vi "Imageprocessing_subVi.vi"(8 "error in (no error)":errorcluster, 10 "Binary Img":T1, 11 "Image In":T1) -> (0 "error out":errorcluster, 3 "Image Dst Out":T1)   [LabVIEW 2020]
doc: "Vi che stima i parametri di calibrazione da un set up specifico (inserire descriz setup!!!).\nCostanti inteerne: Inserire descrizione"
uses:
  <vilib>/vision/Image Controls.llb/IMAQ Image.ctl
  <vilib>/vision/NI_Vision_Development_Module.lvlib
panel:
  in  "stop":bool
  in  "Window Size (32x32)":cluster{"SizeX":i32, "SizeY":i32}={"SizeX"=200, "SizeY"=200}
  in  "Selection Values":T3(array[cluster])=[{"Measurement Parameter"=35, "Range Lower Value"=0.0, "Range Upper Value"=100.0, "Range"=FALSE, "Measurement Type"=FALSE}] {"Measurement Parameter" items=["Center of Mass X", "Center of Mass Y", "First Pixel X", "First Pixel Y", "Bounding Rect Left", "Bounding Rect Top", "Bounding Rect Right", "Bounding Rect Bottom", "Max Feret Diameter Start X", "Max Feret Diameter Start Y", "Max Feret Diameter End X", "Max Feret Diameter End Y", "Max Horiz. Segment Length Left", "Max Horiz. Segment Length Right", "Max Horiz. Segment Length Row", "-", "Bounding Rect Width", "Bounding Rect Height", "Bounding Rect Diagonal", "Perimeter", "Convex Hull Perimeter", "Holes' Perimeter", "Max Feret Diameter", "Equivalent Ellipse Major Axis", "Equivalent Ellipse Minor Axis", "Equivalent Ellipse Minor Axis (Feret)", "Equivalent Rect Long Side", "Equivalent Rect Short Side", "Equivalent Rect Diagonal", "Equivalent Rect Short Side (Feret)", "Average Horiz. Segment Length", "Average Vert. Segment Length", "Hydraulic Radius", "Waddel Disk Diameter", "-", "Area", "Holes' Area", "Particle & Holes' Area", "Convex Hull Area", "Image Area", "-", "Number of Holes", "Number of Horiz. Segments", "Number of Vert. Segments", "-", "Orientation", "Max Feret Diameter Orientation", "-", "% Area/Image Area", "% Area/(Particle & Holes' Area)", "Ratio of Equivalent Ellipse Axes", "Ratio of Equivalent Rect Sides", "-", "Elongation Factor", "Compactness Factor", "Heywood Circularity Factor", "Type Factor", "-", "Sum X", "Sum Y", "Sum XX", "Sum XY", "Sum YY", "Sum XXX", "Sum XXY", "Sum XYY", "Sum YYY", "-", "Moment of Inertia XX", "Moment of Inertia XY", "Moment of Inertia YY", "Moment of Inertia XXX", "Moment of Inertia XXY", "Moment of Inertia XYY", "Moment of Inertia YYY", "Norm. Moment of Inertia XX", "Norm. Moment of Inertia XY", "Norm. Moment of Inertia YY", "Norm. Moment of Inertia XXX", "Norm. Moment of Inertia XXY", "Norm. Moment of Inertia XYY", "Norm. Moment of Inertia YYY", "Hu Moment 1", "Hu Moment 2", "Hu Moment 3", "Hu Moment 4", "Hu Moment 5", "Hu Moment 6", "Hu Moment 7"]}
  out "processed Img":T1(plugin-control)
  out "Image In":T1(plugin-control)
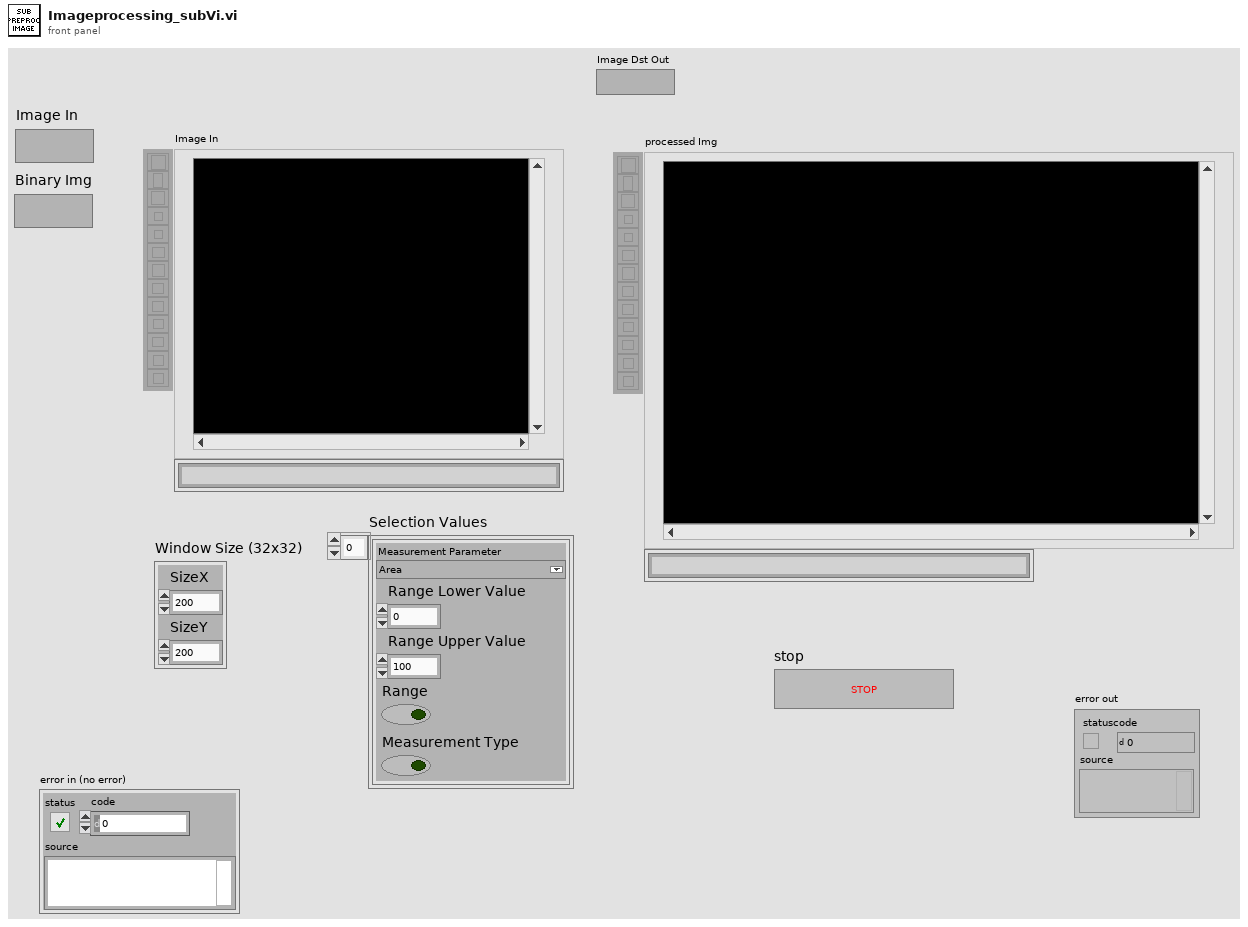
[diagram p1: front panel]
types:
  T1 = typedef "IMAQ Image.ctl" = refnum<image>
  T2 = typedef "Particle Parameters" = i32
  T3 = cluster{"Measurement Parameter":T2, "Range Lower Value":dbl, "Range Upper Value":dbl, "Range":bool, "Measurement Type":bool}[]
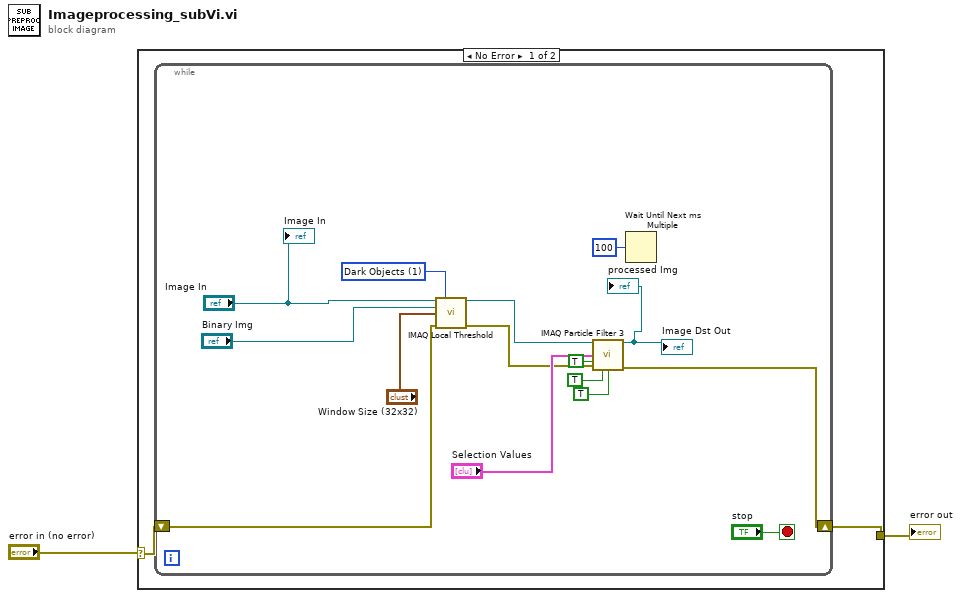
[diagram p0: block diagram]
diagram:
  n1 = case shown="No Error" "error in (no error)" {
    selector: "error in (no error)" -> [w4 w20]
    tunnel: [w3 w20] -> w1
    frame No Error {
      n2 = while {
        shift-right: [w5] -> w3
        shift-left: w4 -> [w11]
        stop <- "stop" stop-if-true
        w18 = u32 1 items=["Bright Objects", "Dark Objects"] ("Look For (Bright Objects)")
        n3 = call "IMAQ Local Threshold"("Image Src"="Image In", "Look For (Bright Objects)"=w18, "Image Dst"="Binary Img", "Window Size (32x32)"="Window Size (32x32)", "error in (no error)"=w11) -> ("Image Dst Out"=w16:T1, "error out"=w10:errorcluster)  [unwired: 9 in]
        n4 = call "IMAQ Particle Filter 3"("Image Src"=w16, "Selection Values"="Selection Values", "Keep/Remove Particles (F)"=TRUE, "error in (no error)"=w10, "Reject Border? (F)"=TRUE, "Fill Holes? (F)"=TRUE) -> ("Image Dst Out"=→"processed Img" →"Image Dst Out":T1, "error out"=w5:errorcluster)  [unwired: 7 in, 1 out]
        n5 = Wait Until Next ms Multiple(millisecond multiple=u32 100) -> ()  [unwired: 1 out]
        "Image In" <- "Image In"
      }
    }
    frame Error {
    }
  }
  "error out" <- w1
